vi "databasedemo.vi"() -> ()   [LabVIEW 2016, in "database.lvlib"]
uses:
  database.lvlib
  <vilib>/addons/database/_DB Variant To Data/Database Variant To Data.xnode
panel:
  in  "data 2":T1
  out "表格控件":string[][](table)
  in  "data":T2 {"单位" items=["ug/L", "mg/L", "ppm", "mg/m3", "cm", "ppb", "ug/m3", "%", "nmol/mol", "umol/mol", "MPN/L", "MPN/100ml", "ng/m3", "NTU", "无量纲", "ms/cm", "us/cm"]}
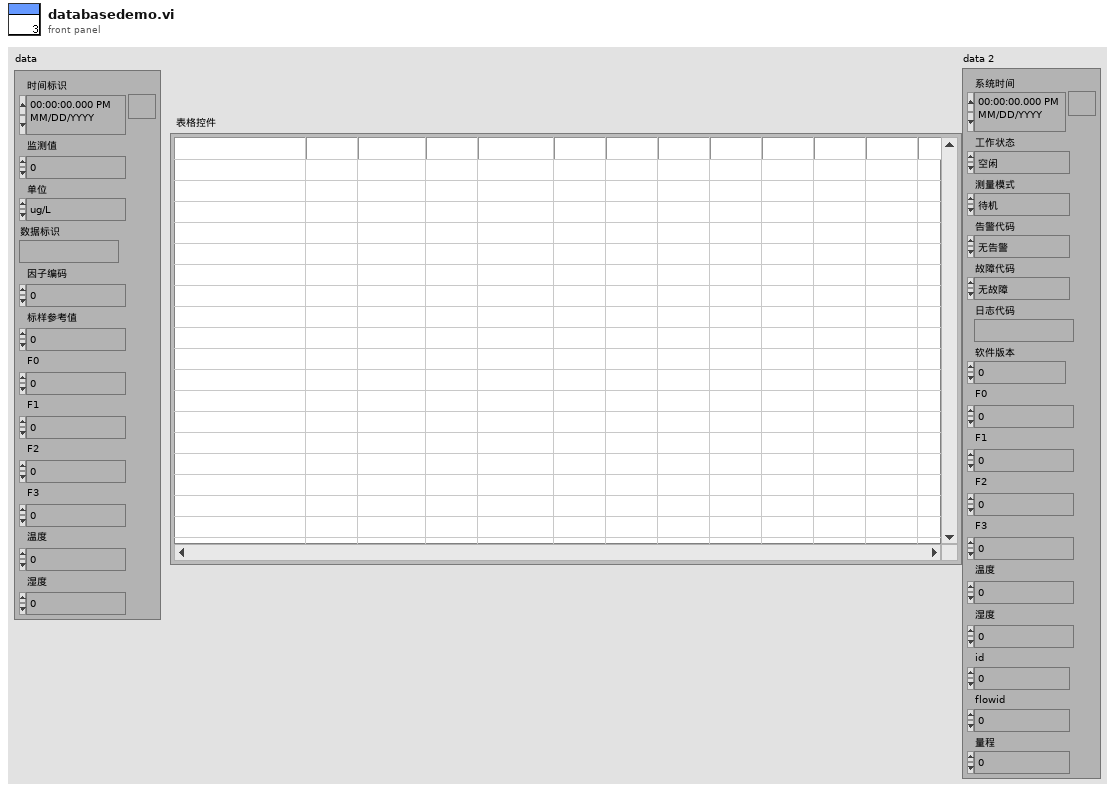
[diagram p1: front panel]
types:
  T1 = cluster{"系统时间":timestamp, "工作状态":enum16{"空闲", "水样测试", "标样核查", "零点核查", "跨度核查", "空白测试", "平行样测试", "加标回收", "空白校准", "标样校准", "初始化（清洗）"}, "测量模式":enum16{"待机", "连续模式", "周期模式", "定点模式", "受控模式", "手动模式"}, "告警代码":enum16{"无告警", "缺试剂告警", "缺水样告警", "缺蒸馏水告警", "缺标液告警", "仪表漏液告警", "标定异常告警", "超量程告警", "加热异常", "低试剂预警", "超上限告警", "超下限告警", "仪表内部其他异常", "滴定异常告警", "电极异常告警", "量程切换告警", "参数设置告警", "PH电极电位异常", "电导率电极异常", "浊度光度异常", "溶解氧电极异常", "溶解氧光强异常", "温度异常告警", "PH异常告警", "溶解氧异常告警", "电导率异常告警", "浊度异常告警", "叶绿素异常告警", "藻密度异常告警", "蓝绿藻异常告警", "ORP异常告警", "氨氮异常告警", "清洁刷异常告警", "SD卡异常告警", "蓝牙异常告警", "Wifi异常告警", "流程异常告警"}, "故障代码":enum16{"无故障", "电机故障", "温度故障", "通讯故障", "滴定故障"}, "日志代码":string, "软件版本":u16, "F0":sgl, "F1":sgl, "F2":sgl, "F3":sgl, "温度":sgl, "湿度":sgl, "id":u16, "flowid":u16, "量程":u16}
  T2 = cluster{"时间标识":timestamp, "监测值":sgl, "单位":u16, "数据标识":string, "因子编码":u32, "标样参考值":sgl, "F0":sgl, "F1":sgl, "F2":sgl, "F3":sgl, "温度":sgl, "湿度":sgl}
  T3 = cluster{"时间标识":timestamp, "测量模式":string, "监测值":sgl, "单位":string, "数据标识":string, "因子编码":string, "标样参考值":sgl, "F0":sgl, "F1":sgl, "F2":sgl, "F3":sgl, "温度":sgl, "湿度":sgl, "量程标识":string}
  T4 = cluster{"系统时间":timestamp, "工作状态":string, "测量模式":string, "告警代码":string, "故障代码":string, "日志代码":string, "软件版本":string, "F0":sgl, "F1":sgl, "F2":sgl, "F3":sgl, "温度":sgl, "湿度":sgl, "id":u16, "flowid":u16, "量程":u16}
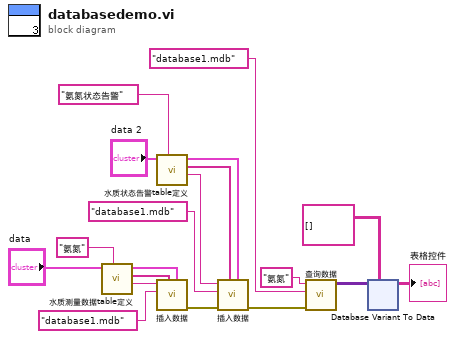
[diagram p0: block diagram]
diagram:
  n1 = call "水质测量数据table定义.vi"("table 输入"="氨氮" ("table"), "data"="data") -> ("table 输出"=w16:string, "columns"=w19:string[], "data输出"=w18:T3)  [unwired: 7 in]
  n2 = call "水质状态告警table定义.vi"("table输入"="氨氮状态告警" ("table"), "data"="data 2") -> ("table输出"=w4:string, "columns"=w5:string[], "data 输出"=w6:T4)  [unwired: 7 in]
  n3 = call "插入数据.vi"("data"=w18, "columns"=w19, "database"="database1.mdb", "table"=w16) -> ("error out"=w8:errorcluster)  [unwired: 7 in]
  n4 = call "插入数据.vi"("data"=w6, "columns"=w5, "error in (no error)"=w8, "database"="database1.mdb", "table"=w4) -> ("error out"=w2:errorcluster)  [unwired: 6 in]
  n5 = call "查询数据.vi"("error in (no error)"=w2, "database"="database1.mdb", "table"="氨氮") -> ("data"=w12:variant[][])  [unwired: 7 in, 1 out]
  n6 = xnode "Database Variant To Data"("database variant"=w12, "type"=string[][] [] ("表格控件")) -> ("data"=→"表格控件":string[][])  [unwired: 1 in, 1 out]
